vi "AES N Teeth M Missing Degrees per Tooth.vi"(7 "NTeeth.Use Cycle? (F)":bool, 9 "Crank.Teeth Duty Cycle":dbl=50.0 caption="NTeeth.Duty Cycle (0 to 100)" min=0.0 max=100.0, 10 "NTeeth.Num Teeth":u16=60) -> (1 "NTeeth.Degrees Low Pulse":fxp<+,60,9> format="%.54g", 2 "NTeeth.Degrees High Pulse":fxp<+,60,9> format="%.54g")   [LabVIEW 2010, in "AES.lvlib" / "AES RT.lvlib"]
doc: "This VI takes the configuration parameters of the crank (Num Teeth and Duty Cycle) in order to calculate the angle in degrees for a single tooth (high pulse) and tooth gap (low pulse) of the crank. The Degrees/high pulse and Degrees/how pulse are then sent to the FPGA to be used by the Crank Angle and Output.vi\n\nNote: Set the \"Use Cycle? (F)\" input to true if your N Teeth M Missing generation loop is referencing the Cycle Angle (0-720) not the Crank Angle (0-360)"
uses:
  AES RT.lvlib
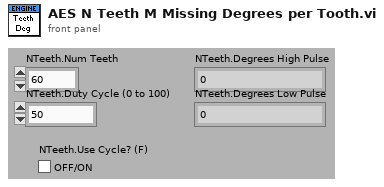
[diagram p1: front panel]
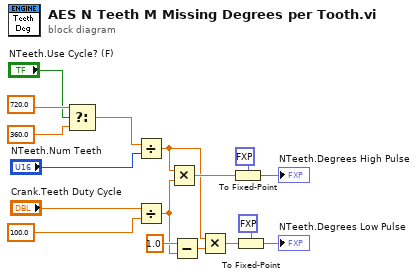
[diagram p0: block diagram]
diagram:
  n1 = Select(t=720.0 ("y"), s="NTeeth.Use Cycle? (F)", f=360.0 ("y")) -> (s? t:f=w3:dbl)
  n2 = Divide(x=w3, y="NTeeth.Num Teeth") -> (x/y=w8:dbl)
  n3 = Divide(x="Crank.Teeth Duty Cycle", y=100.0) -> (x/y=w10:dbl)
  n4 = Multiply(x=w8, y=w10) -> (x*y=w14:dbl)
  n5 = Subtract(x=1.0, y=w10) -> (x-y=w9:dbl)
  n6 = Multiply(x=w8, y=w9) -> (x*y=w7:dbl)
  n7 = To Fixed-Point(fixed-point type=fxp<+,60,9> 0.0 ("Degrees/Tooth"), number=w14) -> (fixed-point=→"NTeeth.Degrees High Pulse":fxp<+,60,9>)
  n8 = To Fixed-Point(fixed-point type=fxp<+,60,9> 0.0 ("Degrees/Tooth"), number=w7) -> (fixed-point=→"NTeeth.Degrees Low Pulse":fxp<+,60,9>)
